vi "Listen & Send Test Cluster Info.vi"() -> ()   [LabVIEW 2017]
uses:
  Common/Typedefs/tagValue.ctl
  Common/Typedefs/command.ctl
  WebSocket.lvclass
panel:
  in  "Send":bool
  in  "Tab Control":T1(tab)
  in  "Tag":string
  in  "Value":string
  in  "Array":string[](array[string])
  in  "Command":string
  in  "Error Code":u32
  in  "Error Message":string
  in  "Type":string(combo)
  out "JSON string":string
  out "trimmed string":string
  out "Rx from Client":string
  out "Headers":variant=variant("Accept-Encoding"=variant(string "gzip, deflate, br"), "Accept-Language"=variant(string "en-US,en;q=0.9"), "Cache-Control"=variant(string "no-cache"), "Connection"=variant(string "Upgrade"), "Host"=variant(string "localhost"), "Origin"=variant(string "http://tattsun.github.io"), "Pragma"=variant(string "no-cache"), "Sec-WebSocket-Extensions"=variant(string "permessage-deflate; client_max_window_bits"), "Sec-WebSocket-Key"=variant(string "dIZ2gIS4iTUMLhpa7t/LlA=="), "Sec-WebSocket-Version"=variant(string "13"), "Upgrade"=variant(string "websocket"), "User-Agent"=variant(string "Mozilla/5.0 (Windows NT 6.1; Win64; x64) AppleWebKit/537.36 (KHTML, like Gecko) Chrome/65.0.3325.181 Safari/537.36"))
  # "Send JSON Message"
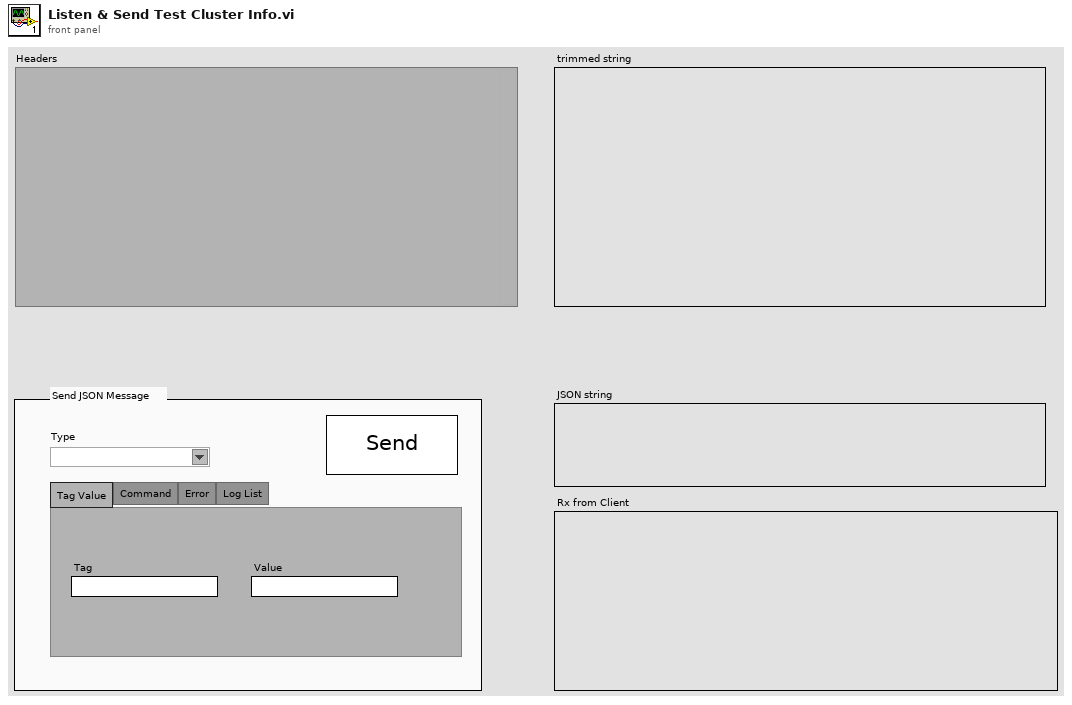
[diagram p1: front panel]
types:
  T1 = enum32{"Tag Value", "Command", "Error", "Log List"}
  T2 = enum16{"Standard", "Buffered", "CRLF", "Immediate"}
  T3 = typedef "tagValue.ctl" = cluster{"type":string, "tag":string, "value":string, "t":string}
  T4 = typedef "command.ctl" = cluster{"type":string, "command":string, "arguments":string[]}
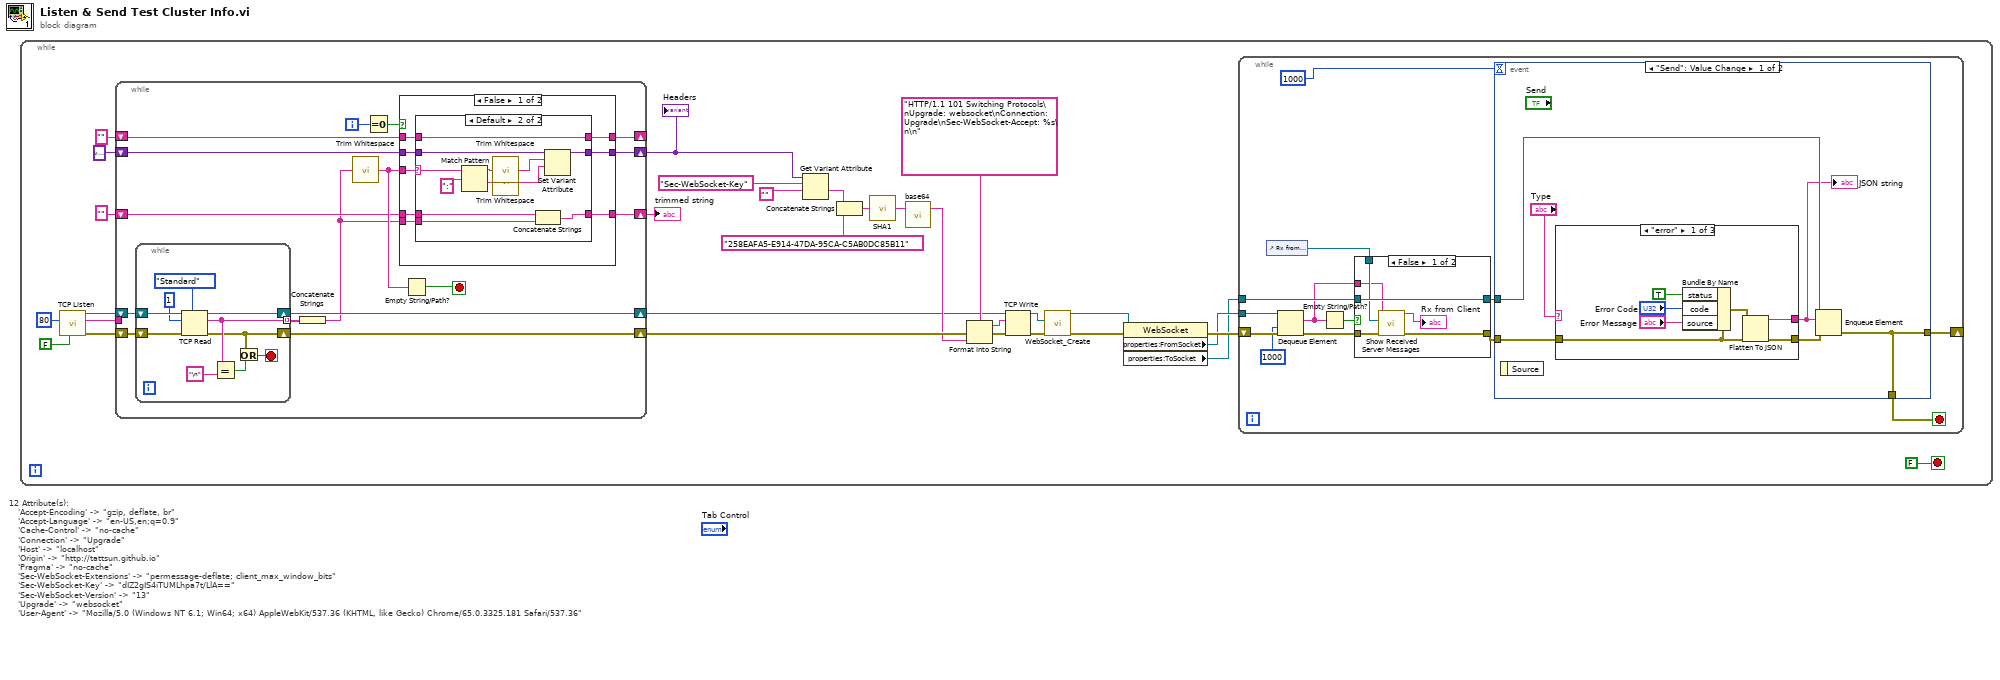
[diagram p0: block diagram]
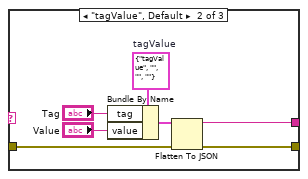
[diagram p3: hidden frame]
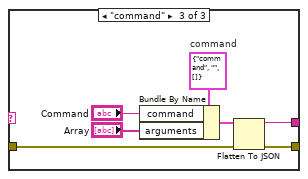
[diagram p4: hidden frame]
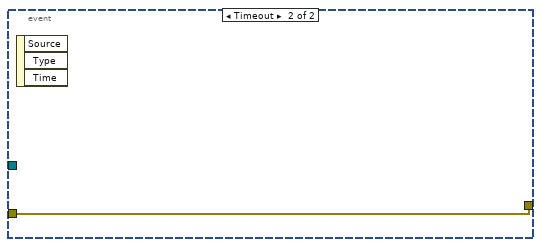
[diagram p5: hidden frame]
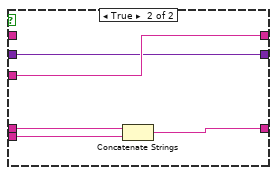
[diagram p7: hidden frame]
diagram:
  # "12 Attribute(s):\n   'Accept-Encoding' -> \"gzip, deflate, br\"\n   'Accept-Language' -> \"en-US,en;q=0.9\"\n   'Cache-Control' -> \"no-cache\"\n   'Connection' -> \"Upgrade\"\n   'Host' -> \"localhost\"\n   'Origin' -> \"http://tattsun.github.io\"\n   'Pragma' -> \"no-cache\"\n   'Sec-WebSocket-Extensions' -> \"permessage-deflate; client_max_window_bits\"\n   'Sec-WebSocket-Key' -> \"dIZ2gIS4iTUMLhpa7t/LlA==\"\n   'Sec-WebSocket-Version' -> \"13\"\n   'Upgrade' -> \"websocket\"\n   'User-Agent' -> \"Mozilla/5.0 (Windows NT 6.1; Win64; x64) AppleWebKit/537.36 (KHTML, like Gecko) Chrome/65.0.3325.181 Safari/537.36\""
  n1 = while {
    stop <- FALSE stop-if-true
    n2 = call <vilib>:"TCP Listen.vi"("resolve remote address (T)"=FALSE, "port"=u16 80) -> ("error out"=w27:errorcluster, "remote address"=w6:string, "connection ID"=w28:refnum<k5>)  [unwired: 5 in, 2 out]
    n3 = while {
      shift-right: [w86] -> w24
      shift-left: variant -> [w87]
      shift-right: [w91] -> _
      shift-left: "" ("trimmed string") -> [w90]
      shift-right: [w85] -> w13
      shift-left: w28 -> [w95]
      shift-right: [w84] -> w21
      shift-left: w27 -> [w94]
      shift-right: [w82] -> w8
      shift-left: "" ("trimmed string") -> [w81]
      tunnel: w6 -> [_]
      i -> [w93]
      stop <- w88 stop-if-true
      n4 = while {
        tunnel: [w100] -> w83 mode=indexing
        shift-right: [w101] -> w85
        shift-left: w95 -> [w105]
        shift-right: [w97] -> w84
        shift-left: w94 -> [w104]
        stop <- w96 stop-if-true
        n5 = TCP Read(connection ID=w105, bytes to read=1, error in (no error)=w104, 7:T2."Standard" ("mode (standard)")) -> (connection ID out=w101:refnum<k5>, data out=w100:string, error out=w97:errorcluster)  [unwired: 1 in]
        n6 = Equal?(x=w100, y="\n") -> (x = y?=w98:bool)
        n7 = Or(x=w97, y=w98) -> (x .or. y?=w96:bool)
      }
      n8 = Concatenate Strings(w83) -> (w80:string)
      n9 = call <vilib>:"Trim Whitespace.vi"("string"=w80) -> ("trimmed string"=w89:string)  [unwired: 1 in]
      n10 = Equal To 0?(x=w93) -> (x = 0?=w92:bool)
      n11 = case shown="False" w92 {
        tunnel: [w109 w133] -> w91
        tunnel: w89 -> [w111 w133]
        tunnel: w90 -> [w110 _]
        tunnel: w87 -> [w113 w132]
        tunnel: [w112 w132] -> w86
        tunnel: w80 -> [w108 w129]
        tunnel: [w107 w130] -> w82
        tunnel: w81 -> [w106 w131]
        frame False {
          n12 = case shown="Default" w111 {
            selector: w111 -> [_ w121]
            tunnel: w113 -> [w116 w125]
            tunnel: [w116 w124] -> w112
            tunnel: w110 -> [w115 w120]
            tunnel: [w115 w120] -> w109
            tunnel: w108 -> [_ w119]
            tunnel: [w114 w118] -> w107
            tunnel: w106 -> [w114 w117]
            frame "" {
            }
            frame Default {
              n13 = Match Pattern(string=w121, regular expression=":" ("trimmed string")) -> (before substring=w126:string, after substring=w127:string)  [unwired: 1 in, 2 out]
              n14 = call <vilib>:"Trim Whitespace.vi"("string"=w126) -> ("trimmed string"=w123:string)  [unwired: 1 in]
              n15 = call <vilib>:"Trim Whitespace.vi"("string"=w127) -> ("trimmed string"=w122:string)  [unwired: 1 in]
              n16 = Concatenate Strings(w117, w119) -> (w118:string)
              n17 = Set Variant Attribute(Variant=w125, name=w123, value=w122) -> (Variant out=w124:variant)  [unwired: 1 in, 2 out]
            }
          }
        }
        frame True {
          n18 = Concatenate Strings(w131, w129) -> (w130:string)
        }
      }
      n19 = Empty String/Path?(string/path=w89) -> (empty?=w88:bool)
    }
    "Headers" <- w24
    "trimmed string" <- w8
    n20 = Get Variant Attribute(Variant=w24, name="Sec-WebSocket-Key" ("trimmed string"), default value (empty Variant)="") -> (value=w20:string)  [unwired: 1 in, 3 out]
    n21 = Concatenate Strings(w20, "258EAFA5-E914-47DA-95CA-C5AB0DC85B11" ("trimmed string")) -> (w19:string)
    n22 = call "SHA1.vi"("String"=w19) -> ("SHA1"=w18:string)
    n23 = call "base64.vi"("string in"=w18) -> ("base64 out"=w17:string)  [unwired: 1 in, 1 out]
    n24 = Format Into String(format string="HTTP/1.1 101 Switching Protocols\nUpgrade: websocket\nConnection: Upgrade\nSec-WebSocket-Accept: %s\n\n" ("trimmed string"), error in=w21, w17) -> (resulting string=w14:string, error out=w15:errorcluster)  [unwired: 1 in]
    n25 = TCP Write(connection ID=w13, data in=w14, error in (no error)=w15) -> (connection ID out=w10:refnum<k5>, error out=w12:errorcluster)  [unwired: 1 in, 1 out]
    n26 = call "WebSocket_Create.vi"("error in (no error)"=w12, "Socket"=w10) -> ("error out"=w11:errorcluster, "reference out"=w4:refnum<class "WebSocket.lvclass">)  [unwired: 8 in]
    n27 = property class="WebSocket"(reference=w4, error in=w11) -> (error out=w5:errorcluster, "properties:FromSocket"=w3:refnum<queue>, "properties:ToSocket"=w2:refnum<queue>)  [unwired: 1 out]
    n28 = while {
      tunnel: w3 -> [w42]
      tunnel: w2 -> [w37]
      shift-right: [w40] -> _
      shift-left: w5 -> [w43]
      stop <- w32 stop-if-true
      n29 = control-ref of="Rx from Client"() -> (w31:refnum<vi>)
      n30 = Dequeue Element(queue=w42, timeout in ms (-1)=1000, error in (no error)=w43) -> (element=w34:string, error out=w38:errorcluster)  [unwired: 2 out]
      n31 = Empty String/Path?(string/path=w34) -> (empty?=w35:bool)
      n32 = case shown="False" w35 {
        tunnel: w38 -> [w48 w51]
        tunnel: [w47 w51] -> w33
        tunnel: w37 -> [w49 w50]
        tunnel: [w49 w50] -> w36
        tunnel: w34 -> [w44 _]
        tunnel: w31 -> [w45 _]
        frame False {
          n33 = call "Show Received Server Messages.vi"("error in (no error)"=w48, "String in"=w45, "Rx String"=w44) -> ("error out"=w47:errorcluster, "Received Messages from RT"=→"Rx from Client":string)  [unwired: 7 in]
        }
        frame True {
        }
      }
      n34 = event shown="[0] \"Send\": Value Change" {
        selector: _ -> [_ _]
        dyn-events: _ -> [_ _]
        timeout: 1000 ("timeout in ms (-1)") -> [_ _]
        tunnel: w36 -> [w57 _]
        tunnel: w33 -> [w56 w79]
        tunnel: [w52 w79] -> w40
        tunnel: [w52 _] -> w32
        event "Send": Value Change {
          n35 = event-data() -> ()  [unwired: 1 in, 1 out]
          n36 = case shown="\"error\"" "Type" {
            tunnel: [w63 w67 w75] -> w55
            tunnel: [w59 w66 w76] -> w54
            tunnel: w56 -> [w58 w65 w72]
            frame "error" {
              n37 = Bundle By Name(cluster=w58, "status"=TRUE, "code"="Error Code", "source"="Error Message") -> (w62:errorcluster)
              n38 = Flatten To JSON(anything=w62, error in (no error)=w58) -> (JSON string=w59:string, 11:w63:errorcluster)  [unwired: 1 in]
            }
            frame "tagValue", Default {
              w68 = T3 {"type"="tagValue", "tag"="", "value"="", "t"=""}  # tagValue
              n39 = Bundle By Name(cluster=w68, "tag"="Tag", "value"="Value") -> (w69:T3)
              n40 = Flatten To JSON(anything=w69, error in (no error)=w65) -> (JSON string=w66:string, 11:w67:errorcluster)  [unwired: 1 in]
            }
            frame "command" {
              w77 = T4 {"type"="command", "command"="", "arguments"=[]}  # command
              n41 = Bundle By Name(cluster=w77, "command"="Command", "arguments"="Array") -> (w78:T4)
              n42 = Flatten To JSON(anything=w78, error in (no error)=w72) -> (JSON string=w76:string, 11:w75:errorcluster)  [unwired: 1 in]
            }
          }
          "JSON string" <- w54
          n43 = Enqueue Element(queue=w57, element=w54, error in (no error)=w55) -> (error out=w52:errorcluster)  [unwired: 1 in, 2 out]
        }
        event Timeout {
          n44 = event-data() -> ()  [unwired: 1 in, 3 out]
        }
      }
    }
  }
